vi "Phasor Explorer Quit Dialog.vi"(9 "App name":string, 11 "PhXP Queue":refnum<queue>) -> (3 "Quit?":bool)   [LabVIEW 2019]
uses:
  SEPXP Q [Element].ctl
  SEPXP Q [Event] List.ctl
  Notebook/Notebook Saved Global.vi
  Notebook/Notebook.lvlib
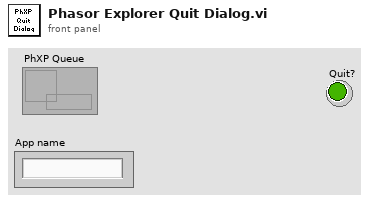
[diagram p1: front panel]
types:
  T1 = typedef "SEPXP Q [Element].ctl" = cluster{"SEPXP Q Event":T2, "Data":variant}
  T2 = typedef "SEPXP Q [Event] List.ctl" = enum16{"Idle", "Initialization", "Show-Hide UC Ticks", "Edit User-defined Gate", "Update Phasor Graph", "Update Sum of Gates Graph", "Update Parameters", "Compute Decay &/or Gates", "Find Pseudo UC Intersections", "Compute alpha(beta) Plot", "Compute Pseudo-Phase Lifetime Plot", "Export Parameters to Clipboard", "Update Phase & Modulus Lifetime", "XY Graph Special Event", "Update Graph Plots Info", "Fit to Circle", "Quit"}
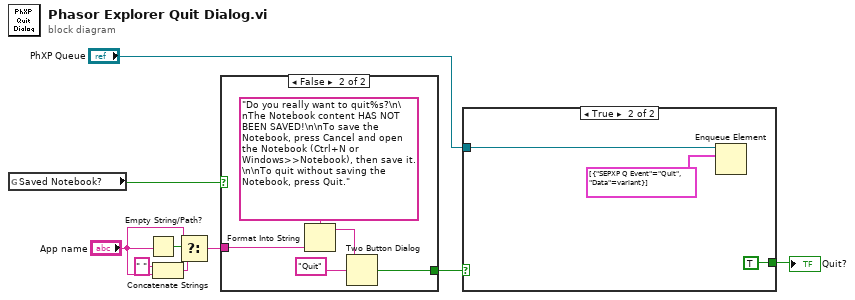
[diagram p0: block diagram]
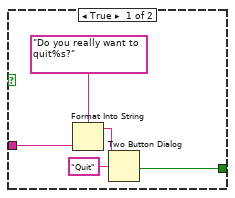
[diagram p2: hidden frame]
diagram:
  n1 = global read "Notebook Saved Global.vi" "Saved Notebook?"() -> (w6:bool)
  n2 = Empty String/Path?(string/path="App name") -> (empty?=w3:bool)
  n3 = Concatenate Strings(" " ("string"), "App name") -> (w4:string)
  n4 = Select(t="App name", s=w3, f=w4) -> (s? t:f=w1:string)
  n5 = case shown="False" w6 {
    tunnel: [w12 w19] -> w8
    tunnel: w1 -> [w10 w15]
    frame True {
      n6 = Format Into String(format string="Do you really want to quit%s?" ("message"), w10) -> (resulting string=w11:string)  [unwired: 2 in, 1 out]
      n7 = Two Button Dialog(message=w11, 2:"Quit" ("T button name (\"OK\")")) -> (T button?=w12:bool)  [unwired: 1 in]
    }
    frame False {
      n8 = Format Into String(format string="Do you really want to quit%s?\n\nThe Notebook content HAS NOT BEEN SAVED!\n\nTo save the Notebook, press Cancel and open the Notebook (Ctrl+N or Windows>>Notebook), then save it.\n\nTo quit without saving the Notebook, press Quit." ("message"), w15) -> (resulting string=w16:string)  [unwired: 2 in, 1 out]
      n9 = Two Button Dialog(message=w16, 2:"Quit" ("T button name (\"OK\")")) -> (T button?=w19:bool)  [unwired: 1 in]
    }
  }
  n10 = case shown="True" w8 {
    tunnel: "PhXP Queue" -> [_ w22]
    tunnel: [_ TRUE ("Discard?")] -> w9
    frame False {
      # "Cancel"
    }
    frame True {
      n11 = Enqueue Element(queue=w22, element=T1[] [{"SEPXP Q Event"=enum."Quit", "Data"=variant}]) -> ()  [unwired: 2 in, 3 out]
    }
  }
  "Quit?" <- w9
